vi "Enclose in Structure - Look Up Structure.vi"() -> (3 "Found Obj Ref":refnum<vi>)   [LabVIEW 2020]
uses:
  <vilib>/Platform/TimedLoop/XDataNode/wakeup.ctl
  <vilib>/Platform/TimedLoop/XDataNode/XDNodeRunTimeDep.lvlib
  <vilib>/Platform/TimedLoop/XDataNode/nitl_modes.ctl
  <vilib>/Platform/TimedLoop/XDataNode/timing_clust.ctl
  <vilib>/platform/TimedLoop/XDataNode/XDataNode.xnode
  <vilib>/Utility/traverseref.llb/TRef TravTarget.ctl
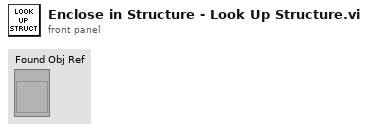
[diagram p1: front panel]
types:
  T1 = typedef "TRef TravTarget.ctl" = enum16{"FP", "BD", "Other"}
  T2 = typedef "XDNodeRunTimeDep.lvlib/timing_clust.ctl" = cluster{"Expected End [f-1]":u64, "Actual End [f-1]":u64, "Finished Late? [f-1]":bool, "Expected End [i-1]":u64, "Actual End [i-1]":u64, "Finished Late? [i-1]":bool, "Expected Start [i]":u64, "Actual Start [i]":u64, "Expected Start [f]":u64, "Actual Start [f]":u64, "Source Name":string, "Structure Name":string, "Period":i64, "Deadline":i64, "Offset":i64, "Start":i64, "Priority":i32, "Timeout":i32, "Mode":T3, "Wakeup Reason":T4, "Error":errorcluster, "Source Type":string, "Secondary Source Type":string, "Global End Time":u64, "Global Start Time":u64, "Frame Duration":u64, "Iteration Duration":u64, "Assigned CPU":i32, "I/O Scan Engine Mode":u32}
  T3 = typedef "XDNodeRunTimeDep.lvlib/nitl_modes.ctl" = enum32{"No Change", "Process missed periods, maintain original phase", "Discard missed periods, maintain original phase", "Process missed periods, ignore original phase", "Discard missed periods, ignore original phase"}
  T4 = typedef "XDNodeRunTimeDep.lvlib/wakeup.ctl" = enum32{"Normal", "Aborted", "Asynchronous wakeup", "Timing source error", "Timed loop error", "Timeout"}
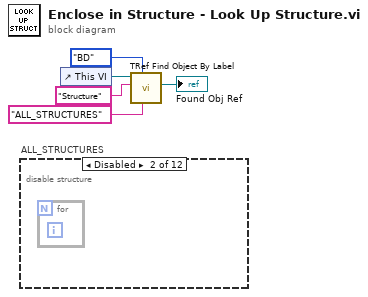
[diagram p0: block diagram]
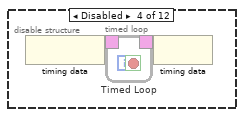
[diagram p4: hidden frame]
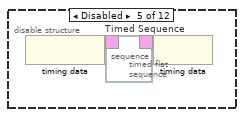
[diagram p5: hidden frame]
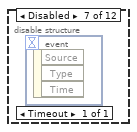
[diagram p8: hidden frame]
diagram:
  n1 = disable-structure "ALL_STRUCTURES" shown="Disabled" {
    frame Enabled {
    }
    frame Disabled {
      n2 = for {
      }
    }
    frame Disabled {
      n3 = while {
        stop <- _ stop-if-true
      }
    }
    frame Disabled {
      n4 = node-c288() -> (w7:T2)
      n5 = timed-loop "Timed Loop" {
        timing: w7 -> [_]
        timing-out: [_] -> w6
        stop <- _ stop-if-true
      }
      n6 = node-c288(w6) -> ()
    }
    frame Disabled {
      n7 = node-c288() -> (w13:T2)
      n8 = timed-sequence "Timed Sequence" {
        timing: w13 -> [_]
        timing-out: [_] -> w12
        n9 = timed-flat-sequence {
        }
      }
      n10 = node-c288(w12) -> ()
    }
    frame Disabled {
      n11 = case shown="True" {
        selector: _ -> [_ _]
        frame False {
        }
        frame True {
        }
      }
    }
    frame Disabled {
      n12 = event shown="[0] Timeout" {
        selector: _ -> [_]
        dyn-events: _ -> [_]
        timeout: _ -> [_]
        event Timeout {
          n13 = event-data() -> ()  [unwired: 1 in, 3 out]
        }
      }
    }
    frame Disabled {
      n14 = in-place "In Place Element Structure" {
      }
    }
    frame Disabled {
      n15 = flat-sequence {
        frame #0 {
        }
      }
    }
    frame Disabled {
      n16 = disable-structure "Diagram Disable Structure" shown="Disabled" {
        frame Disabled {
        }
        frame Enabled {
        }
      }
    }
    frame Disabled {
      n17 = disable-structure "Conditional Disable Structure" shown="Default" {
        frame Enabled {
        }
      }
    }
    frame Disabled {
      n18 = disable-structure "Type Specialization Structure" shown="[0] Accepted" {
        frame Enabled {
        }
        frame Disabled {
        }
      }
    }
  }
  n19 = control-ref of="This VI"() -> (w5:refnum<vi>)
  n20 = call <vilib>:"TRef Find Object By Label.vi"("Label"="ALL_STRUCTURES", "Traverse Target"=TRef_TravTarget."BD", "Class Name"="Structure", "VI Ref"=w5) -> ("Found Obj Ref"=→"Found Obj Ref":refnum<vi>)  [unwired: 4 in, 3 out]
